vi "CreateUserEventRef.vi"(9 "Label.Text":string, 10 "referenceToEventRef":refnum<vi>) -> (3 "UserEventCtlRef":refnum<vi>)   [LabVIEW 2024, in "AddNewEvent.lvlib"]
doc: "Move the control into a event refnum constant"
uses:
  Event/AddNewEvent.lvlib
  <vilib>/Utility/miscctls.llb/LVPositionTypeDef.ctl
  EventRefTemplate.vi
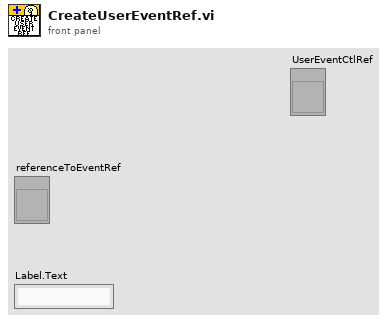
[diagram p1: front panel]
types:
  T1 = typedef "LVPositionTypeDef.ctl" = cluster{"Left":i32, "Top":i32}
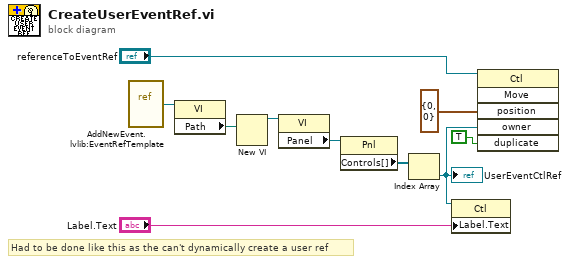
[diagram p0: block diagram]
diagram:
  # "Had to be done like this as the can't dynamically create a user ref"
  n1 = vi-ref "AddNewEvent.lvlib:EventRefTemplate.vi"() -> (w1:refnum<vi>)
  n2 = property class="VI"(reference=w1) -> ("Path"=w6:path)  [unwired: 1 in, 2 out]
  n3 = New VI(10:w6) -> (3:w5:refnum<vi>)  [unwired: 6 in, 1 out]
  n4 = property class="VI"(reference=w5) -> ("Panel"=w10:refnum<vi>)  [unwired: 1 in, 2 out]
  n5 = property class="Pnl"(reference=w10) -> ("Controls[]"=w7:refnum<vi>[])  [unwired: 1 in, 2 out]
  n6 = Index Array(array=w7) -> (element=w4:refnum<vi>)  [unwired: 1 in]
  "UserEventCtlRef" <- w4
  n7 = property class="Ctl"(reference=w4, "Label.Text"="Label.Text") -> ()  [unwired: 1 in, 2 out]
  n8 = invoke class="Ctl" method="Move"(reference="referenceToEventRef", "position"=T1 {"Left"=0, "Top"=0}, "owner"=w4, "duplicate"=TRUE ("Duplicate? (F)")) -> ()  [unwired: 2 in, 6 out]
